vi "Initialize.vi"(8 "error in (no error)":errorcluster, 11 "NXP in":refnum<class "NXP.lvclass">) -> (0 "error out":errorcluster, 3 "NXP out":refnum<class "NXP.lvclass">)   [LabVIEW 2019, in "NXP.lvclass"]
uses:
  NXP.lvclass
  C:/Users/Luis/Documents/Ingenieria/Git_versiones/PROYECTO-FINAL-INSTRUMENTACI-N-VIRTUAL/Clase Padre/Serial Device.lvclass
  Clase Padre/Serial Device.lvclass/Serial Device.ctl
  <vilib>/Instr/_visa.llb/VISA Configure Serial Port (Instr).vi
  Clase Padre/Serial Device.lvclass
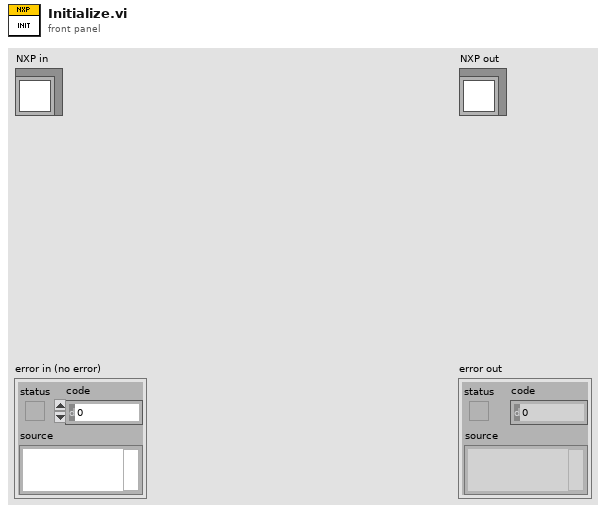
[diagram p1: front panel]
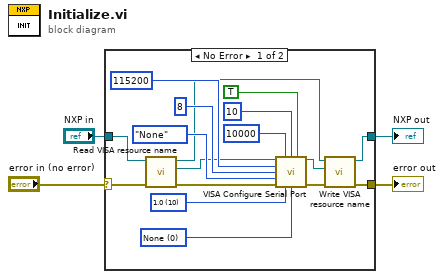
[diagram p0: block diagram]
diagram:
  n1 = case shown="No Error" "error in (no error)" {
    selector: "error in (no error)" -> [w6 w23]
    tunnel: [w10 w23] -> w2
    tunnel: [w12 w22] -> w3
    tunnel: "NXP in" -> [w9 w22]
    frame No Error {
      w14 = u16 0 items=["None", "XON/XOFF", "RTS/CTS", "XON/XOFF & RTS/CTS", "DTR/DSR", "XON/XOFF & DTR/DSR"] ("flow control (0:none)")
      w15 = u16 10 items=["1.0"=10, "1.5"=15, "2.0"=20] ("stop bits (10: 1 bit)")
      n2 = call "Read VISA resource name.vi"("error in (no error)"=w6, "Serial Device in"=w9) -> ("error out"=w5:errorcluster, "VISA resource name"=w7:refnum<visa-resource-name>, "Serial Device out"=w8:refnum<class "NXP.lvclass">)  [unwired: 7 in]
      n3 = call-poly "VISA Configure Serial Port"("VISA resource name"=w7, "timeout (10sec)"=u32 10000, "termination char\n(0xA = '\\n' = LF)"=u8 10 ("termination char\n(0xA = '\\n' = LF)"), "Enable Termination\nChar (T)"=TRUE ("Enable Termination\nChar (T)"), "baud rate (9600)"=u32 115200, "data bits (8)"=u16 8, "parity (0:none)"=enum16{"None", "Odd", "Even", "Mark", "Space"}."None", "error in (no error)"=w5, "stop bits (10: 1 bit)"=w15, "flow control (0:none)"=w14) -> ("VISA resource name out"=w13:refnum<visa-resource-name>, "error out"=w11:errorcluster)  [unwired: 4 in]
      n4 = call "Write VISA resource name.vi"("error in (no error)"=w11, "VISA resource name"=w13, "Serial Device in"=w8) -> ("error out"=w10:errorcluster, "Serial Device out"=w12:refnum<class "NXP.lvclass">)  [unwired: 7 in]
    }
    frame Error {
    }
  }
  "error out" <- w2
  "NXP out" <- w3
